vi "Graph loeschen.vi"(8 "Fehler (Eingang, kein Fehler)":errorcluster, 10 "Ergebnis  Array in":refnum<vi>[](array[refnum]), 11 "Graph":refnum<vi>[](array[refnum])) -> (0 "Fehler (Ausgang)":errorcluster, 2 "Ergebnis  Array out":refnum<vi>[](array[refnum]), 3 "Graph out":refnum<vi>[](array[refnum]))   [LabVIEW 2020, in "EPA 1065.lvlib" / "HovaCAL Interference verificaton.lvlib"]
uses:
  HovaCAL Interference verificaton.lvlib
  Messdaten/Aktionen FGV Messdaten.ctl
  Messdaten/Messdaten.lvlib
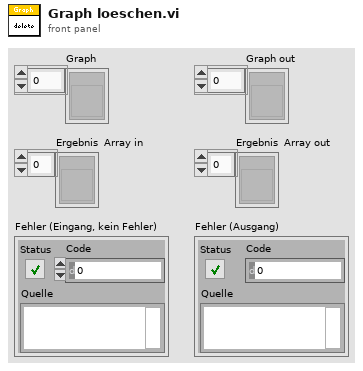
[diagram p1: front panel]
types:
  T1 = typedef "Messdaten.lvlib/Aktionen FGV Messdaten.ctl" = enum16{"lesen", "schreiben", "löschen", "Mittelwerte", "Komponente"}
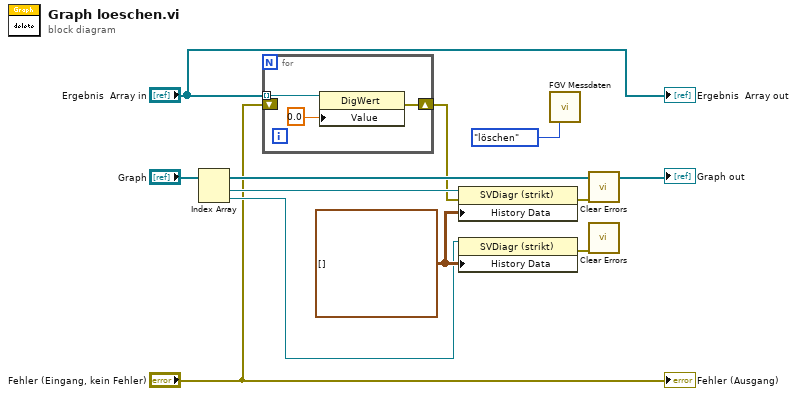
[diagram p0: block diagram]
diagram:
  w9 = waveform(dbl)[][] [] ("Historiendaten")
  n1 = Index Array(array="Graph") -> (element #1=w5:refnum<vi>, element #2=w4:refnum<vi>)  [unwired: 2 in]
  n2 = for {
    tunnel: "Ergebnis  Array in" -> [w13] mode=indexing
    shift-right: [w11] -> w1
    shift-left: "Fehler (Eingang, kein Fehler)" -> [_]
    n3 = property class="DigWert"(reference=w13, "Value"=0.0 ("Y-Achse.Bereich:Minimum")) -> (error out=w11:errorcluster)  [unwired: 1 in, 1 out]
  }
  n4 = property on="Eigenschaftsknoten" class="SVDiagr (strikt)"(reference=w5, error in=w1, "History Data"=w9) -> (error out=w10:errorcluster)  [unwired: 1 out]
  n5 = property on="Eigenschaftsknoten" class="SVDiagr (strikt)"(reference=w4, "History Data"=w9) -> (error out=w7:errorcluster)  [unwired: 1 in, 1 out]
  n6 = call "FGV Messdaten.vi"("Aktionen"=Aktionen_FGV_Messdaten."löschen") -> ()  [unwired: 6 in, 9 out]
  n7 = call <vilib>:"Clear Errors.vi"("error in (no error)"=w10) -> ()  [unwired: 5 in, 2 out]
  n8 = call <vilib>:"Clear Errors.vi"("error in (no error)"=w7) -> ()  [unwired: 5 in, 2 out]
  "Fehler (Ausgang)" <- "Fehler (Eingang, kein Fehler)"
  "Graph out" <- "Graph"
  "Ergebnis  Array out" <- "Ergebnis  Array in"
